vi "KeepAliveUDP.vi"(11 "FPGA in":refnum<queue>) -> (3 "FPGA out":refnum<queue>)   [LabVIEW 2019, in "FPGA.lvlib"]
uses:
  FPGA.lvlib
  FPGA.ctl
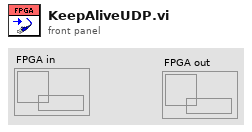
[diagram p1: front panel]
types:
  T1 = typedef "FPGA.lvlib/FPGA.ctl" = cluster{"Start freq. [Hz]":dbl, "Sweep duration [s]":dbl, "Freq. step [Hz]":dbl, "DAC Sample Rate":dbl, "ADC Sample Rate":dbl, "CMD port":u16, "DFAST port":u16, "CMD ID":refnum<k16>, "DFAST ID":refnum<k16>, "CMD error out":errorcluster, "FPGA IP":string, "DFAST error out ":errorcluster, "Stop freq. [Hz]":dbl, "Discrete sweep":bool, "Initial NCO":u32, "Difference NCO":i32, "step NCO":i64, "Final NCO":u32, "clocks for step":u32, "demodulation":bool, "NCO Phase Precision":u32, "NCO Sample Rate":dbl, "Time for step [s]":dbl, "NCO freq. resolution":dbl, "Sweep speed [Hz/s]":dbl, "Connected":bool, "Slew Rate [V/us]":dbl, "Parameters_ok":bool, "Amplitude [mVpp]":dbl, "Scale Factor":fxp<+,16,0>, "Acquiring":bool, "DAC-ADC Latency":u16, "Digital Gain":i32, "Number of steps":i32, "Averaging preferred":bool, "Filter Order":u32, "Settling":enum16{"99%", "99,9%"}}
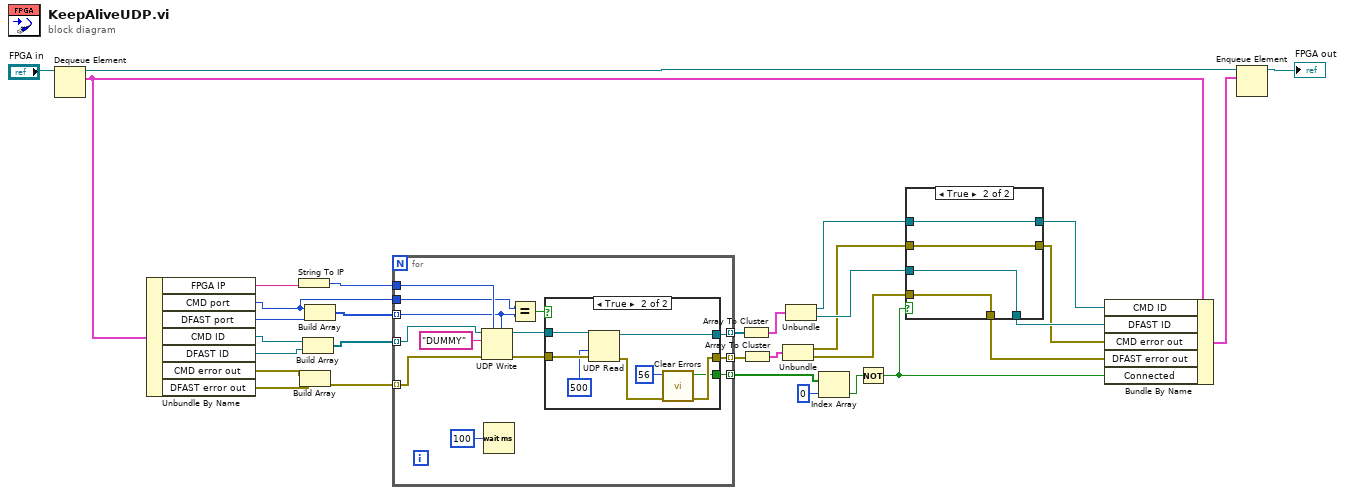
[diagram p0: block diagram]
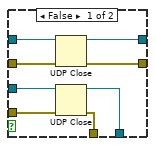
[diagram p2: hidden frame]
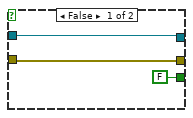
[diagram p3: hidden frame]
diagram:
  n1 = Dequeue Element(queue="FPGA in") -> (queue out=w24:refnum<queue>, element=w22:T1)  [unwired: 2 in, 2 out]
  n2 = Unbundle By Name(w22) -> ("FPGA IP"=w28:string, "CMD port"=w13:u16, "DFAST port"=w32:u16, "CMD ID"=w20:refnum<k16>, "DFAST ID"=w19:refnum<k16>, "CMD error out"=w21:errorcluster, "DFAST error out"=w30:errorcluster)
  n3 = String To IP(1:w28) -> (0:w31:u32)
  n4 = Build Array(w21, w30) -> (w29:errorcluster[])
  n5 = Build Array(w20, w19) -> (w18:refnum<k16>[])
  n6 = Build Array(w13, w32) -> (w23:u16[])
  n7 = for {
    tunnel: [w38] -> w17 mode=indexing
    tunnel: w31 -> [w45]
    tunnel: [w37] -> w16 mode=indexing
    tunnel: w29 -> [w42] mode=indexing
    tunnel: w23 -> [w34] mode=indexing
    tunnel: w18 -> [w41] mode=indexing
    tunnel: w13 -> [w35]
    tunnel: [w33] -> w11 mode=indexing
    n8 = UDP Write(address=w45, port or service name=w34, connection ID=w41, data in="DUMMY", 8:w42) -> (error out=w39:errorcluster, 3:w40:refnum<k16>)  [unwired: 1 in]
    n9 = Wait (ms)(milliseconds to wait=u32 100) -> ()  [unwired: 1 out]
    n10 = Equal?(x=w35, y=w34) -> (x = y?=w36:bool)
    n11 = case shown="True" w36 {
      tunnel: w40 -> [w48 w55]
      tunnel: w39 -> [w47 w54]
      tunnel: [w48 w53] -> w38
      tunnel: [w47 w51] -> w37
      tunnel: [FALSE ("specific error cleared?") w50] -> w33
      frame False {
      }
      frame True {
        n12 = UDP Read(connection ID=w55, timeout ms (25000)=500, 8:w54) -> (error out=w52:errorcluster, 3:w53:refnum<k16>)  [unwired: 1 in, 3 out]
        n13 = call <vilib>:"Clear Errors.vi"("error in (no error)"=w52, "specific error code to clear (0: all)"=56) -> ("error out"=w51:errorcluster, "specific error cleared?"=w50:bool)  [unwired: 4 in]
      }
    }
  }
  n14 = Array To Cluster(array=w17) -> (cluster=w15:cluster{"[0]":refnum<k16>, "[1]":refnum<k16>})
  n15 = Array To Cluster(array=w16) -> (cluster=w14:cluster{"[0]":errorcluster, "[1]":errorcluster})
  n16 = Unbundle(w14) -> ("[0]"=w4:errorcluster, "[1]"=w2:errorcluster)
  n17 = Unbundle(w15) -> ("[0]"=w9:refnum<k16>, "[1]"=w8:refnum<k16>)
  n18 = Index Array(array=w11, index=0) -> (element=w10:bool)
  n19 = Not(x=w10) -> (.not. x?=w5:bool)
  n20 = case shown="True" w5 {
    tunnel: w9 -> [w64 w68]
    tunnel: w8 -> [w63 w67]
    tunnel: [w62 w67] -> w7
    tunnel: [w61 w68] -> w6
    tunnel: w4 -> [w60 w66]
    tunnel: [w59 w66] -> w3
    tunnel: w2 -> [w58 w65]
    tunnel: [w57 w65] -> w1
    frame False {
      n21 = UDP Close(connection ID=w64, 8:w60) -> (connection ID out=w61:refnum<k16>, error out=w59:errorcluster)
      n22 = UDP Close(connection ID=w63, 8:w58) -> (connection ID out=w62:refnum<k16>, error out=w57:errorcluster)
    }
    frame True {
    }
  }
  n23 = Bundle By Name(cluster=w22, "CMD ID"=w6, "DFAST ID"=w7, "CMD error out"=w3, "DFAST error out"=w1, "Connected"=w5) -> (w25:T1)
  n24 = Enqueue Element(queue=w24, element=w25) -> (queue out=→"FPGA out":refnum<queue>)  [unwired: 2 in, 2 out]
